vi "Handle Trigger Channel.vi"(8 "error in (no error)":errorcluster, 9 "Trigger Type":T1, 10 "TDMS datalogger configuration":refnum<class "TDMS datalogger configuration.lvclass">, 11 "engine configuration in":refnum<class "engine configuration.lvclass">) -> (0 "error out":errorcluster, 1 "trigger channel name":string, 2 "TDMS datalogger configuration out":refnum<class "TDMS datalogger configuration.lvclass">, 3 "engine configuration out":refnum<class "engine configuration.lvclass">)   [LabVIEW 2015, in "TDMS datalogger editor node.lvclass"]
uses:
  TDMS datalogger editor node.lvclass
  module/configuration/TDMS datalogger configuration.lvclass
  module/configuration/Trigger Type.ctl
  <vilib>/NI/Module Execution Interface/Engine Configuration/engine configuration.lvclass
  <vilib>/NI/Configuration Framework/serializable configuration/NISE_CEF_serializable configuration.lvclass/NISE_CEF_serializable configuration.ctl
  <vilib>/Utility/LVClass/Get LV Class Name.vi
  <vilib>/NI/Configuration Framework/error generator/NISE_error generator.vi
  <vilib>/NI/Configuration Framework/serializable configuration/NISE_CEF_serializable configuration.lvclass
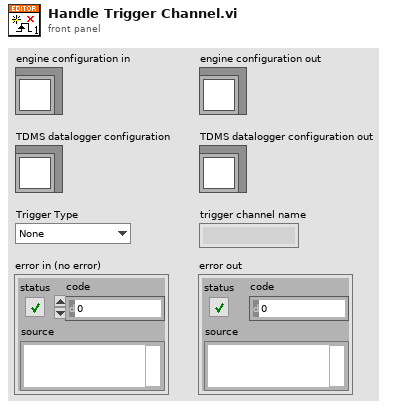
[diagram p1: front panel]
types:
  T1 = typedef "TDMS datalogger configuration.lvclass/Trigger Type.ctl" = enum16{"None", "Start"}
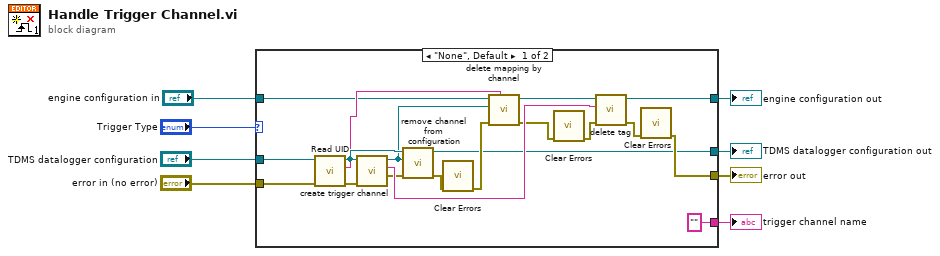
[diagram p0: block diagram]
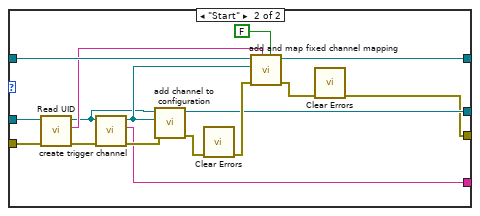
[diagram p2: hidden frame]
diagram:
  n1 = case shown="\"None\", Default" "Trigger Type" {
    tunnel: [w14 w43] -> w2
    tunnel: "engine configuration in" -> [w13 w40]
    tunnel: [w15 w29] -> w5
    tunnel: "error in (no error)" -> [w11 w36]
    tunnel: "TDMS datalogger configuration" -> [w12 w31]
    tunnel: [w10 w30] -> w7
    tunnel: ["" ("trigger channel name") w28] -> w8
    frame "None", Default {
      n2 = call <vilib>:"Read UID.vi"("error in"=w11, "configuration in"=w12) -> ("error out"=w24:errorcluster, "instance id"=w25:string, "configuration out"=w26:refnum<class "TDMS datalogger configuration.lvclass">)  [unwired: 7 in]
      n3 = call "create trigger channel.vi"("error in"=w24, "TDMS datalogger configuration"=w26) -> ("error out"=w16:errorcluster, "trigger channel name"=w27:string, "enable channel"=w17:refnum<class "TBM channel.lvclass">)  [unwired: 7 in]
      n4 = call "remove channel from configuration.vi"("error in"=w16, "TBM channel in"=w17, "TDMS datalogger configuration in"=w26) -> ("error out"=w22:errorcluster, "TDMS datalogger configuration out"=w10:refnum<class "TDMS datalogger configuration.lvclass">)  [unwired: 7 in]
      n5 = call <vilib>:"Clear Errors.vi"("error in (no error)"=w22) -> ("error out"=w23:errorcluster)  [unwired: 5 in, 1 out]
      n6 = call <vilib>:"delete mapping by channel.vi"("owner ID"=w25, "error in"=w23, "channel"=w17, "engine configuration in"=w13) -> ("error out"=w20:errorcluster, "engine configuration out"=w18:refnum<class "engine configuration.lvclass">)  [unwired: 6 in]
      n7 = call <vilib>:"Clear Errors.vi"("error in (no error)"=w20) -> ("error out"=w19:errorcluster)  [unwired: 5 in, 1 out]
      n8 = call <vilib>:"delete tag.vi"("error in"=w19, "tag name"=w27, "engine configuration in"=w18) -> ("error out"=w21:errorcluster, "engine configuration out"=w14:refnum<class "engine configuration.lvclass">)  [unwired: 7 in]
      n9 = call <vilib>:"Clear Errors.vi"("error in (no error)"=w21) -> ("error out"=w15:errorcluster)  [unwired: 5 in, 1 out]
    }
    frame "Start" {
      n10 = call <vilib>:"Read UID.vi"("error in"=w36, "configuration in"=w31) -> ("error out"=w35:errorcluster, "instance id"=w34:string, "configuration out"=w32:refnum<class "TDMS datalogger configuration.lvclass">)  [unwired: 7 in]
      n11 = call "create trigger channel.vi"("error in"=w35, "TDMS datalogger configuration"=w32) -> ("error out"=w42:errorcluster, "trigger channel name"=w28:string, "enable channel"=w41:refnum<class "TBM channel.lvclass">)  [unwired: 7 in]
      n12 = call "add channel to configuration.vi"("error in"=w42, "TBM channel in"=w41, "TDMS datalogger configuration in"=w32) -> ("error out"=w38:errorcluster, "TDMS datalogger configuration out"=w30:refnum<class "TDMS datalogger configuration.lvclass">)  [unwired: 7 in]
      n13 = call <vilib>:"Clear Errors.vi"("error in (no error)"=w38) -> ("error out"=w37:errorcluster)  [unwired: 5 in, 1 out]
      n14 = call <vilib>:"add and map fixed channel mapping.vi"("set module as owner"=FALSE, "module instance"=w34, "error in"=w37, "fixed channel"=w41, "engine configuration in"=w40) -> ("error out"=w39:errorcluster, "engine configuration out"=w43:refnum<class "engine configuration.lvclass">)  [unwired: 5 in]
      n15 = call <vilib>:"Clear Errors.vi"("error in (no error)"=w39) -> ("error out"=w29:errorcluster)  [unwired: 5 in, 1 out]
    }
  }
  "trigger channel name" <- w8
  "TDMS datalogger configuration out" <- w7
  "error out" <- w5
  "engine configuration out" <- w2
